vi "run_holding_noise.vi"(8 "error in":errorcluster, 9 "data in":T1={"daq_ao 1"="Dev1/ao0", "daq_ai 1"="Dev1/ai0", "experiment day folder"=path "D:/DATA/8-27-15 save func testing/test.lvm", "Multiclamp init error"=0, "Multiclamp Handle Out"=0, "sampling rate (Hz)"=10000, "trial name"=""}, 10 "holding time (s)":dbl=1.0, 11 "controls array in":refnum<vi>[](array[refnum])) -> (0 "error out":errorcluster, 1 "data out":T1={"daq_ao 1"="Dev1/ao0", "daq_ai 1"="Dev1/ai0", "experiment day folder"=path "D:/DATA/8-27-15 save func testing/test.lvm", "Multiclamp init error"=0, "Multiclamp Handle Out"=0, "sampling rate (Hz)"=10000, "trial name"=""}, 2 "cell quality bad":bool, 3 "controls array out":refnum<vi>[](array[refnum]))   [LabVIEW 2019]
uses:
  wc_protocol_v1.003 Folder/whole_cell_protocol/Controls/cell_stats-v02.ctl
  Controls/Data.ctl
  get_data_from_control_memtest.vi
panel:
  out "data out (pA or mV)":waveform(dbl)[](graph)
  out "Time has Elapsed":bool
  out "cell stats":T2 {"STD" format="%010.2f"; "Variance" format="%010.2f"; "Rt (MOhms)" format="%010.2f"; "tau (ms)" format="%08.2g"; "Cm (pF)" format="%08.2f"; "Ra (MOhms)" format="%010.2f"; "Rm (MOhms)" format="%010.2f"; "Ihold (pA)" format="%010.2f"}
  out "view memtest":waveform(dbl)(graph)
  # "RUN_HOLDING"
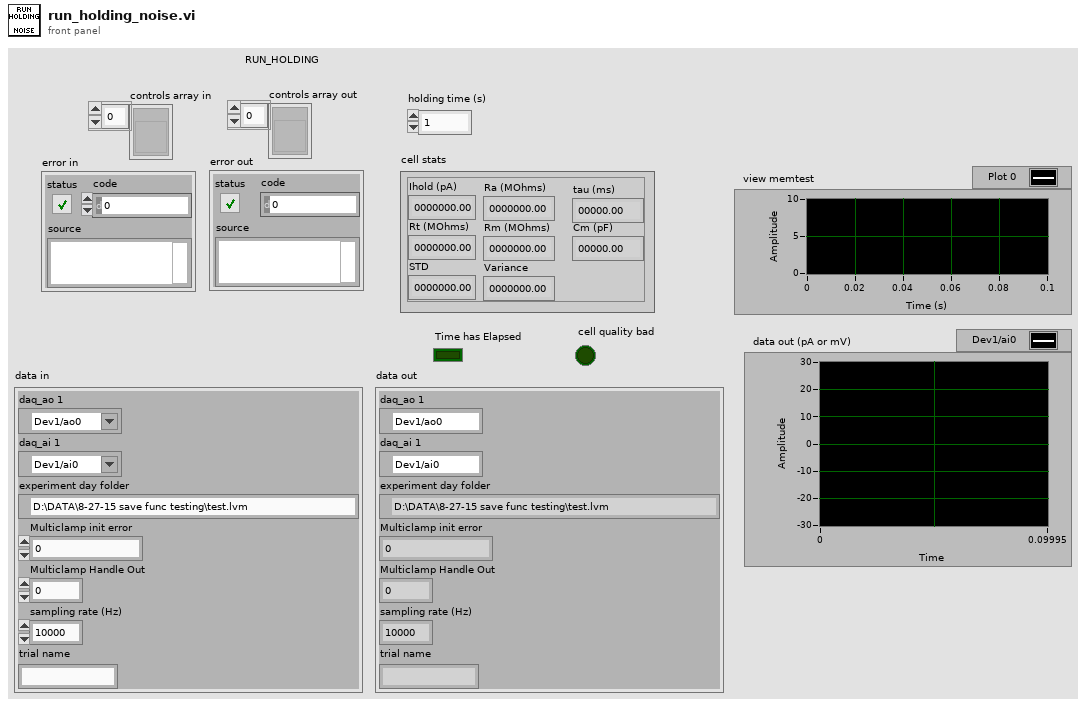
[diagram p1: front panel]
types:
  T1 = typedef "Data.ctl" = cluster{"daq_ao 1":tag, "daq_ai 1":tag, "experiment day folder":path, "Multiclamp init error":i32, "Multiclamp Handle Out":u32, "sampling rate (Hz)":i32, "trial name":string}
  T2 = typedef "cell_stats-v02.ctl" = cluster{"Ihold (pA)":dbl, "Rm (MOhms)":dbl, "Ra (MOhms)":dbl, "Cm (pF)":dbl, "tau (ms)":dbl, "Rt (MOhms)":dbl, "Variance":dbl, "STD":dbl}
  T3 = typedef "memtest_def.ctl" = cluster{"Samples to Read":i32, "Rate (Hz)":dbl, "Amplitude (mV/pA)":dbl, "Offset (mV/pA)":dbl, "Frequency (Hz)":dbl, "duty cycle (%)":dbl, "phase":dbl}
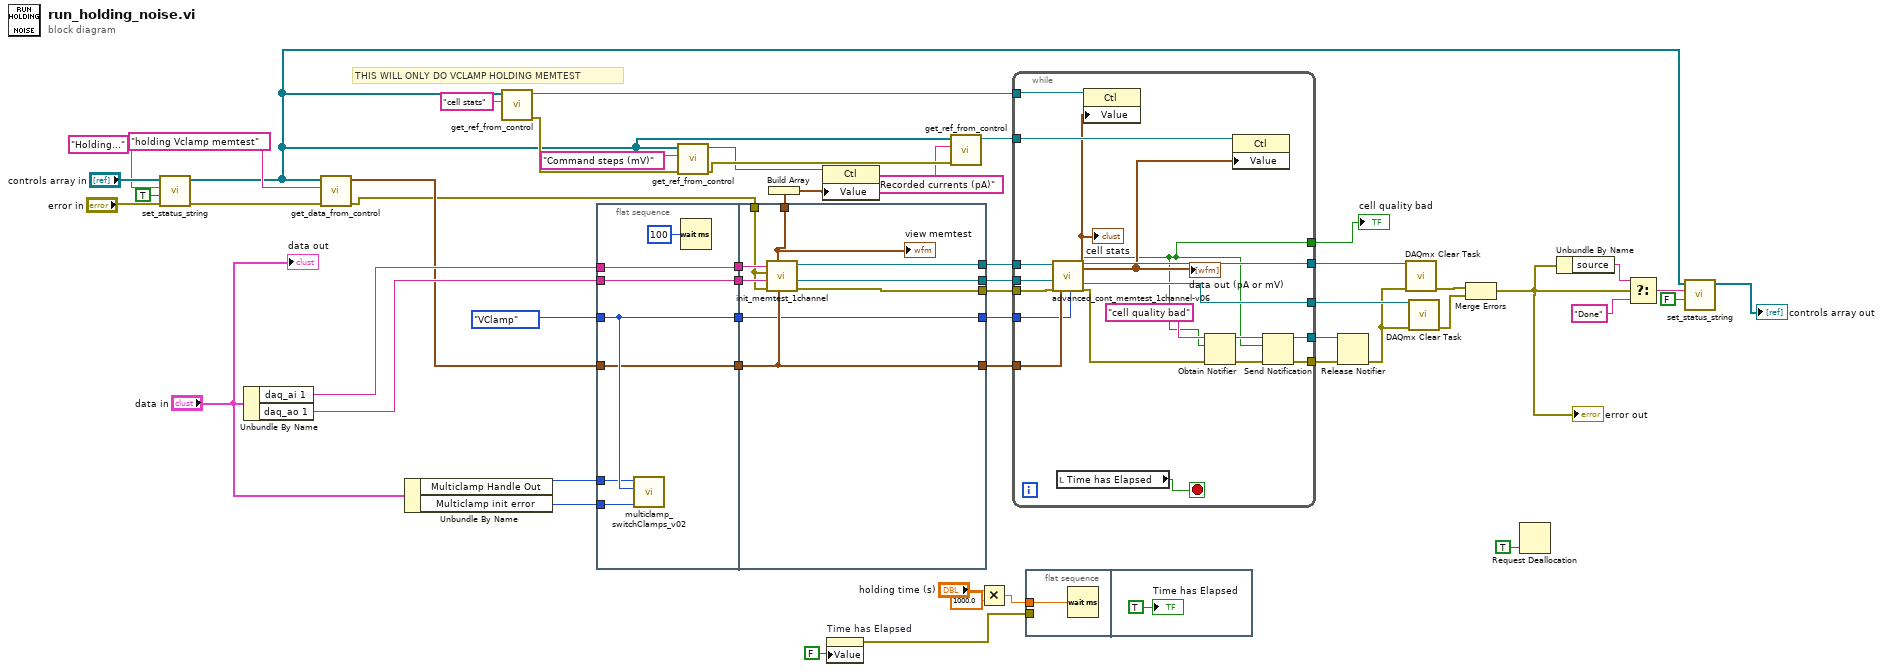
[diagram p0: block diagram]
diagram:
  # "THIS WILL ONLY DO VCLAMP HOLDING MEMTEST"
  n1 = call "set_status_string.vi"("error in"="error in", "new line?"=TRUE, "status string in"="Holding...", "controls array"="controls array in") -> ("error out"=w23:errorcluster, "controls array out"=w17:refnum<vi>[])  [unwired: 6 in]
  n2 = Unbundle By Name("data in") -> ("daq_ai 1"=w42:tag, "daq_ao 1"=w41:tag)
  n3 = call-poly "get_data_from_control.vi"("error in"=w23, "control label"="holding Vclamp memtest", "controls array"=w17) -> ("error out"=w33:errorcluster, "memtest output"=w37:T3)  [unwired: 7 in]
  n4 = Unbundle By Name("data in") -> ("Multiclamp Handle Out"=w39:u32, "Multiclamp init error"=w40:i32)
  n5 = call "get_ref_from_control.vi"("control label"="cell stats", "controls array"=w17) -> ("error out"=w19:errorcluster, "reference out"=w34:refnum<vi>)  [unwired: 8 in]
  n6 = flat-sequence {
    tunnel: [w60] -> w54
    tunnel: w42 -> [w60]
    tunnel: w41 -> [w59]
    tunnel: [w59] -> w53
    tunnel: enum16{"VClamp", "IClamp"}."VClamp" ("which clamp") -> [w58]
    tunnel: [w58] -> w51
    tunnel: w39 -> [w57]
    tunnel: w40 -> [w56]
    tunnel: [w55] -> w50
    tunnel: w37 -> [w55]
    tunnel: w54 -> [w70]
    tunnel: w53 -> [w69]
    tunnel: w51 -> [w64]
    tunnel: w50 -> [w66]
    tunnel: [w68] -> w49
    tunnel: [w67] -> w48
    tunnel: [w66] -> w47
    tunnel: [w65] -> w46
    tunnel: [w64] -> w45
    tunnel: w33 -> [w63]
    tunnel: [w62] -> w12
    frame #0 {
      n7 = call "multiclamp_switchClamps_v02.vi"("error in"=w56, "which clamp"=w58, "Multiclamp Handle in"=w57) -> ()  [unwired: 7 in, 2 out]
      n8 = Wait (ms)(milliseconds to wait=u32 100) -> ()  [unwired: 1 out]
    }
    frame #1 {
      n9 = call "init_memtest_1channel.vi"("memtest"=w66, "AO error in"=w63, "AO physical channels"=w69, "AI error in"=w63, "AI Physical Channels"=w70) -> ("AO error out"=w65:errorcluster, "AO task out"=w67:refnum<k21>, "AI task out"=w68:refnum<k21>, "view memtest"=w62:waveform(dbl))  [unwired: 2 in, 1 out]
      "view memtest" <- w62
    }
  }
  n10 = call "get_ref_from_control.vi"("error in"=w19, "control label"="Command steps (mV)", "controls array"=w17) -> ("error out"=w18:errorcluster, "reference out"=w14:refnum<vi>)  [unwired: 7 in]
  n11 = Build Array(w12) -> (w13:waveform(dbl)[])
  n12 = property class="Ctl"(reference=w14, "Value"=w13) -> ()  [unwired: 1 in, 2 out]
  n13 = property on="Time has Elapsed" class="Bool (strict)"("Value"=FALSE ("Time has Elapsed")) -> (error out=w8:errorcluster)  [unwired: 2 in, 1 out]
  n14 = call "get_ref_from_control.vi"("error in"=w18, "control label"="Recorded currents (pA)", "controls array"=w17) -> ("reference out"=w20:refnum<vi>)  [unwired: 7 in, 1 out]
  n15 = Multiply(x="holding time (s)", y=1000.0) -> (x*y=w9:dbl)
  n16 = while {
    tunnel: w49 -> [w89]
    tunnel: w48 -> [w88]
    tunnel: w47 -> [w87]
    tunnel: w46 -> [w86]
    tunnel: w45 -> [w85]
    tunnel: [w84] -> w44
    tunnel: [w83] -> w43
    tunnel: [w72] -> w4
    tunnel: w34 -> [w81]
    tunnel: w20 -> [w80]
    tunnel: [w75] -> w7
    tunnel: [w71] -> w5
    stop <- w82 stop-if-true
    n17 = call "advanced_cont_memtest_1channel-v06.vi"("Pulse AI task in"=w89, "Pulse AO task in"=w88, "error in"=w86, "memtest"=w87, "which clamp"=w85) -> ("Pulse AI task out"=w84:refnum<k21>, "data out (pA or mV)"=w79:waveform(dbl)[], "cell stats"=w78:T2, "cont memtest error?"=w75:bool, "Pulse AO task out"=w83:refnum<k21>, "error out"=w74:errorcluster)  [unwired: 6 in, 3 out]
    "cell stats" <- w78
    "data out (pA or mV)" <- w79
    n18 = local read "Time has Elapsed"() -> (w82:bool)
    n19 = property class="Ctl"(reference=w81, "Value"=w78) -> ()  [unwired: 1 in, 2 out]
    n20 = Obtain Notifier(name (unnamed)="cell quality bad", notification data type=w75, error in (no error)=w74) -> (notifier out=w76:refnum<notifier>, error out=w73:errorcluster)  [unwired: 1 in, 1 out]
    n21 = property class="Ctl"(reference=w80, "Value"=w79) -> ()  [unwired: 1 in, 2 out]
    n22 = Send Notification(notification=w75, notifier=w76, error in (no error)=w73) -> (notifier out=w71:refnum<notifier>, error out=w72:errorcluster)
  }
  "cell quality bad" <- w7
  n23 = flat-sequence {
    tunnel: w9 -> [w90]
    tunnel: w8 -> [_]
    frame #0 {
      n24 = Wait (ms)(milliseconds to wait=w90) -> ()  [unwired: 1 out]
    }
    frame #1 {
      "Time has Elapsed" <- TRUE ("Time has Elapsed")
    }
  }
  n25 = Release Notifier(notifier=w5, error in (no error)=w4) -> (error out=w2:errorcluster)  [unwired: 1 in, 2 out]
  n26 = call <vilib>:"DAQmx Clear Task.vi"("task in"=w44, "error in"=w2) -> ("error out"=w32:errorcluster)  [unwired: 13 in]
  n27 = call <vilib>:"DAQmx Clear Task.vi"("task in"=w43, "error in"=w2) -> ("error out"=w31:errorcluster)  [unwired: 13 in]
  n28 = Merge Errors(w32, w31) -> (w6:errorcluster)
  "error out" <- w6
  n29 = Request Deallocation(TRUE ("flag")) -> ()
  n30 = Unbundle By Name(w6) -> ("source"=w28:string)
  n31 = Select(t=w28, s=w6, f="Done") -> (s? t:f=w29:string)
  n32 = call "set_status_string.vi"("new line?"=FALSE, "status string in"=w29, "controls array"=w17) -> ("controls array out"=→"controls array out":refnum<vi>[])  [unwired: 7 in, 1 out]
  "data out" <- "data in"
